vi "tm_deinitialize.vi"(8 "error in (no error)":errorcluster {"code" format="%.0x"}) -> (0 "error out":errorcluster {"code" format="%.0x"})   [LabVIEW 2015]
uses:
  tmcamcon.dll
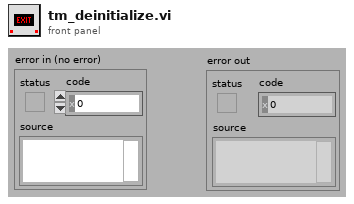
[diagram p1: front panel]
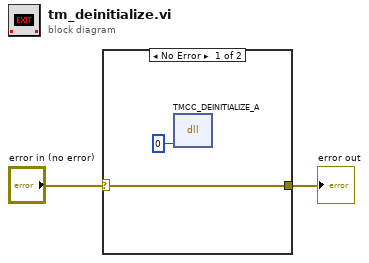
[diagram p0: block diagram]
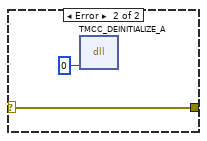
[diagram p2: hidden frame]
diagram:
  n1 = case shown="No Error" "error in (no error)" {
    selector: "error in (no error)" -> [w4 w6]
    tunnel: [w4 w6] -> w2
    frame No Error {
      n2 = dll-call lib="tmcamcon.dll" fn="TMCC_DEINITIALIZE_A"("force"=0) -> ()  [unwired: 5 in, 2 out]
    }
    frame Error {
      n3 = dll-call lib="tmcamcon.dll" fn="TMCC_DEINITIALIZE_A"("force"=0) -> ()  [unwired: 5 in, 2 out]
    }
  }
  "error out" <- w2
